vi "MC scan tcp timeout message.vi"() -> (3 "Which Button?":T1(ring)=enum."Center Button")   [LabVIEW 2018]
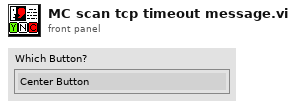
[diagram p1: front panel]
types:
  T1 = enum16{"Left Button", "Center Button", "Right Button", "Window Close"}
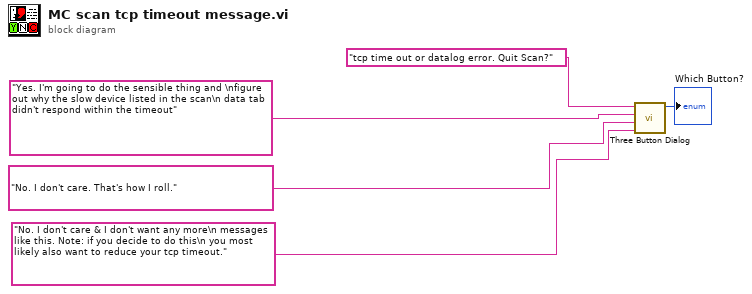
[diagram p0: block diagram]
diagram:
  n1 = call <vilib>:"Three Button Dialog.vi"("Right Button Text (\"Cancel\")"="No. I don't care & I don't want any more\n messages like this. Note: if you decide to do this\n you most likely also want to reduce your tcp timeout." ("F button name (\"Cancel\")"), "Center Button Text (\"No\")"="No. I don't care. That's how I roll." ("F button name (\"Cancel\")"), "Left Button Text (\"Yes\")"="Yes. I'm going to do the sensible thing and \nfigure out why the slow device listed in the scan\n data tab didn't respond within the timeout" ("T button name (\"OK\")"), "message"="tcp time out or datalog error. Quit Scan?" ("T button name (\"OK\")")) -> ("Which Button?"=→"Which Button?":T1)  [unwired: 7 in]
